vi "EVM_Sweep_record_ALL.vi"() -> ()   [LabVIEW 2023, in "EVM.lvlib"]
uses:
  EVM.lvlib
  Clover_Cell.lvlib
  lib/Keysight/Keysight.lvlib
panel:
  in  "Air_Loss":dbl=8.0
  in  "Cable_Loss":dbl=8.0
  in  "WaitingTime(ms)":u32=1000
  in  "FileNote":string
  in  "TRXmode":u16(ring)=1 items=["QUERY_TELEM_2 (V)"=2, "QUERY_TELEM_1 (H)"=1]
  out "SG Power (dBm)":i32
  in  "Stop Power":i32=8
  in  "Start Power":i32=-40
  in  "SG":refnum<visa-resource-name>="TCPIP0::192.168.100.200::inst0::INSTR"
  in  "SA":refnum<visa-resource-name>="TCPIP0::192.168.100.230::inst0::INSTR"
  in  "AvgTimes":i32=5
  out "Spectrum Data":dbl[](graph)
  out "AiP_8":dbl format="%#2.2f"
  out "AiP_7":dbl format="%#2.2f"
  out "AiP_6":dbl format="%#2.2f"
  out "AiP_5":dbl format="%#2.2f"
  out "AiP_4":dbl format="%#2.2f"
  out "AiP_3":dbl format="%#2.2f"
  out "AiP_2":dbl format="%#2.2f"
  out "AiP_1":dbl format="%#2.2f"
  # "Temperature"
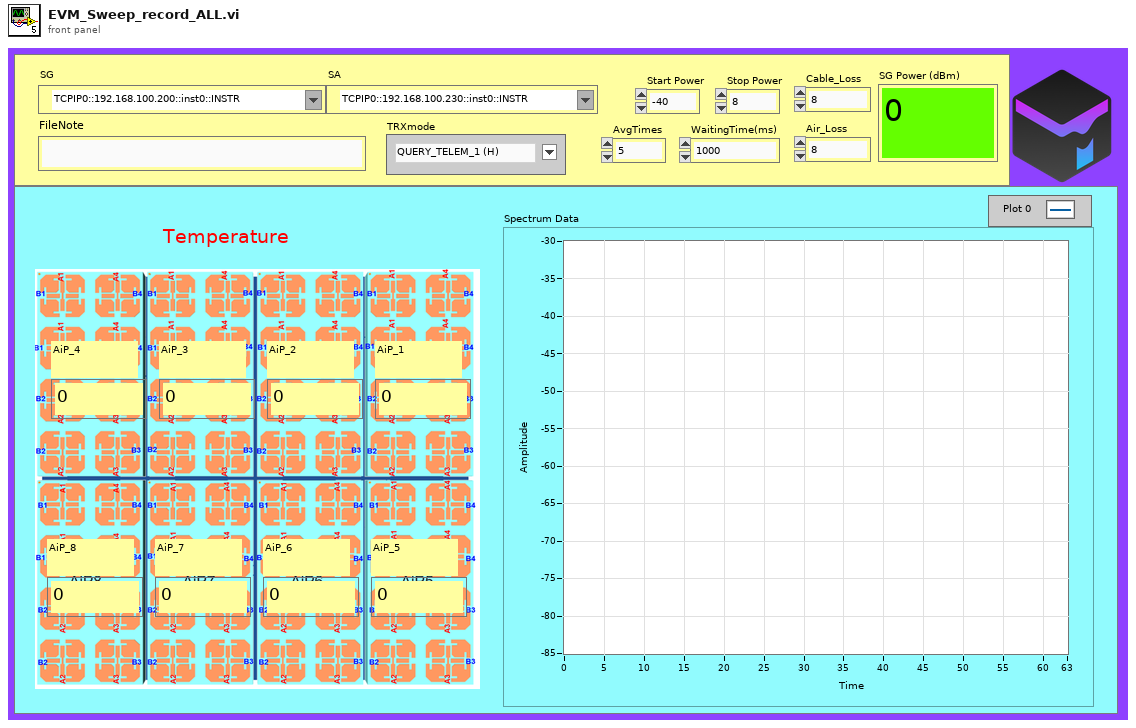
[diagram p1: front panel]
types:
  T1 = cluster{"RMS EVM Avg (dB)":dbl, "RMS EVM Avg (%)":dbl, "Frequency Error Avg (Hz)":dbl, "Avg Burst Power Avg (dBm)":dbl, "Frequency Error Avg (ppm)":dbl}
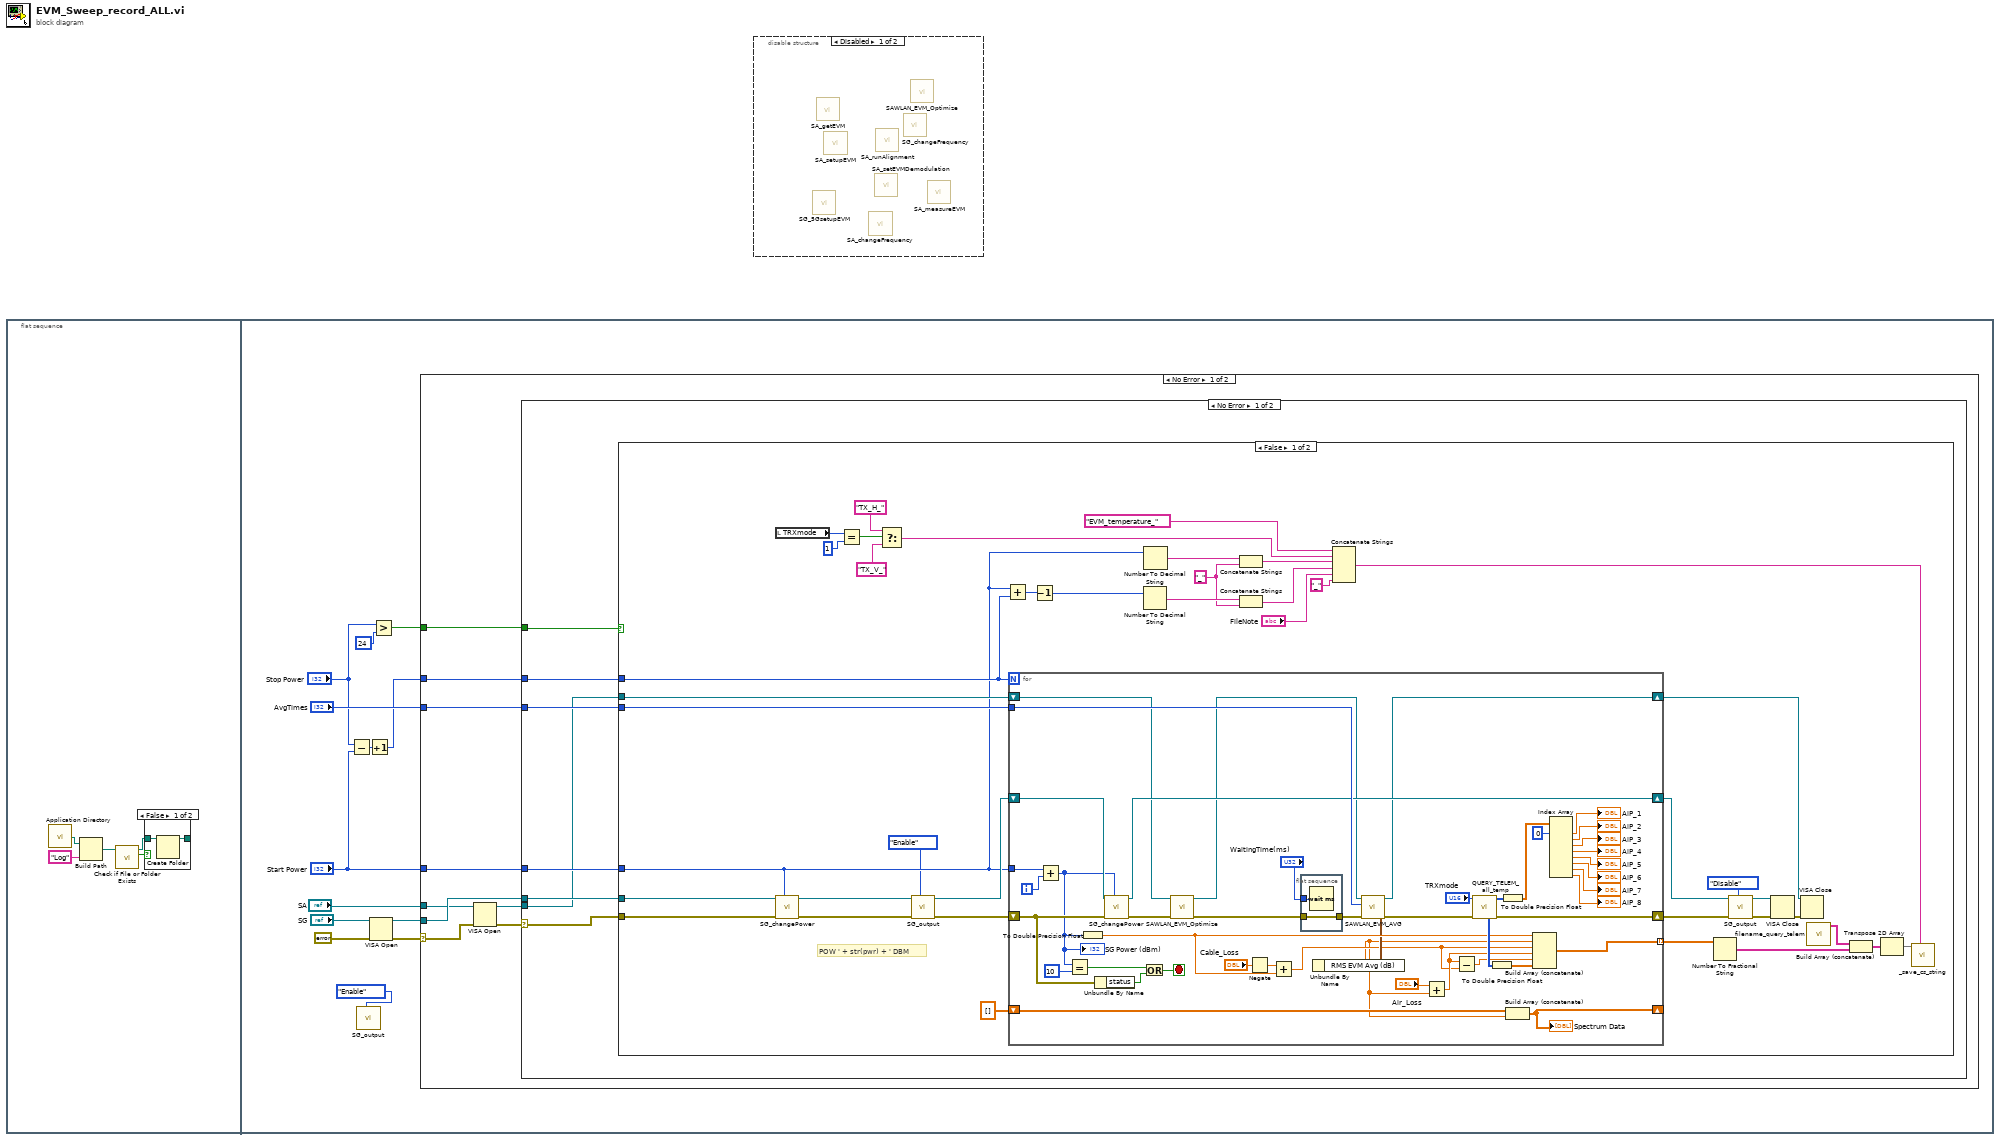
[diagram p0: block diagram]
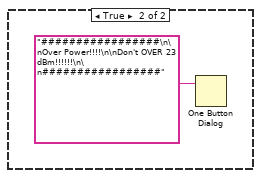
[diagram p4: hidden frame]
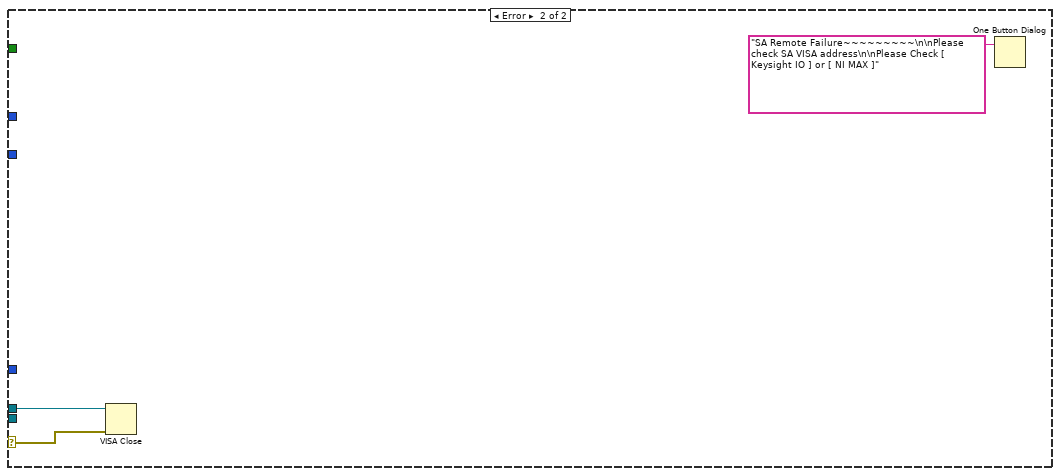
[diagram p5: hidden frame]
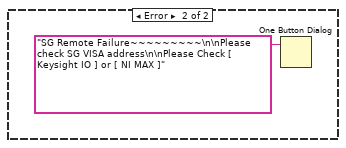
[diagram p6: hidden frame]
diagram:
  n1 = flat-sequence {
    frame #0 {
      n2 = call <vilib>:"Application Directory.vi"() -> ("Application Directory"=w4:path)
      n3 = Build Path(base path=w4, name or relative path="Log") -> (appended path=w1:path)
      n4 = call <vilib>:"Check if File or Folder Exists.vi"("path"=w1) -> ("file or folder exists?"=w3:bool, "dup path"=w2:path)  [unwired: 8 in, 1 out]
      n5 = case shown="False" w3 {
        tunnel: w2 -> [w7 w8]
        tunnel: [w6 w8] -> _
        frame False {
          n6 = Create Folder(path (use dialog)=w7) -> (created path=w6:path)  [unwired: 2 in, 2 out]
        }
        frame True {
        }
      }
    }
    frame #1 {
      n7 = Subtract(x="Stop Power", y="Start Power") -> (x-y=w18:i32)
      n8 = call "SG_output.vi"("Func."=enum16{"Disable", "Enable"}."Enable") -> ()  [unwired: 9 in, 2 out]
      n9 = Increment(x=w18) -> (x+1=w17:i32)
      n10 = VISA Open(error in (no error)=errorcluster {"status"=FALSE, "code"=0, "source"=""}, VISA resource name="SG") -> (VISA resource name=w12:refnum<visa-resource-name>, error out=w10:errorcluster)  [unwired: 3 in]
      n11 = Greater?(x="Stop Power", y=24) -> (0:w21:bool)
      n12 = case shown="No Error" w10 {
        selector: w10 -> [w23 _]
        tunnel: w21 -> [w30 _]
        tunnel: "Start Power" -> [w29 _]
        tunnel: "AvgTimes" -> [w28 _]
        tunnel: w17 -> [w27 _]
        tunnel: w12 -> [w26 _]
        tunnel: "SA" -> [w25 _]
        frame No Error {
          n13 = VISA Open(error in (no error)=w23, VISA resource name=w25) -> (VISA resource name=w24:refnum<visa-resource-name>, error out=w22:errorcluster)  [unwired: 3 in]
          n14 = case shown="No Error" w22 {
            selector: w22 -> [w31 w128]
            tunnel: w30 -> [w37 _]
            tunnel: w29 -> [w36 _]
            tunnel: w28 -> [w35 _]
            tunnel: w27 -> [w34 _]
            tunnel: w26 -> [w33 w129]
            tunnel: w24 -> [w32 _]
            frame No Error {
              n15 = case shown="False" w37 {
                tunnel: w35 -> [w78 _]
                tunnel: w36 -> [w40 _]
                tunnel: w31 -> [w76 _]
                tunnel: w33 -> [w75 _]
                tunnel: w34 -> [w73 _]
                tunnel: w32 -> [w49 _]
                frame False {
                  w65 = "_"
                  # "POW ' + str(pwr) + ' DBM"
                  n16 = local read "TRXmode"() -> (w48:u16)
                  n17 = call "SG_changePower.vi"("dBm"=w40, "error in"=w76, "VISA in"=w75) -> ("error out"=w77:errorcluster, "VISA out"=w74:refnum<visa-resource-name>)  [unwired: 6 in, 1 out]
                  n18 = Equal?(x=w48, y=u16 1) -> (x = y?=w46:bool)
                  n19 = Select(t="TX_H_" ("delimiter (\\t)"), s=w46, f="TX_V_" ("delimiter (\\t)")) -> (s? t:f=w43:string)
                  n20 = call "SG_output.vi"("Func."=enum16{"Disable", "Enable"}."Enable", "error in"=w77, "VISA in"=w74) -> ("error out"=w71:errorcluster, "VISA out"=w72:refnum<visa-resource-name>)  [unwired: 7 in]
                  n21 = Add(x=w40, y=w73) -> (x+y=w69:i32)
                  n22 = for {
                    N: w73 -> [_]
                    tunnel: w78 -> [w124]
                    tunnel: w40 -> [w122]
                    tunnel: [w121] -> w57 mode=indexing
                    shift-right: [w118] -> w70
                    shift-left: w71 -> [w102]
                    shift-right: [w115] -> w62
                    shift-left: w72 -> [w114]
                    shift-right: [w98] -> w50
                    shift-left: w49 -> [w81]
                    shift-right: [w94] -> _
                    shift-left: dbl[] [] -> [w95]
                    i -> [w123]
                    stop <- w101 stop-if-true
                    n23 = Add(x=w122, y=w123) -> (x+y=w84:i32)
                    "SG Power (dBm)" <- w84
                    n24 = Equal?(x=w84, y=10) -> (x = y?=w100:bool)
                    n25 = To Double Precision Float(number=w84) -> (double precision float=w91:dbl)
                    n26 = Unbundle By Name(w102) -> ("status"=w99:bool)
                    n27 = call "SG_changePower.vi"("dBm"=w84, "error in"=w102, "VISA in"=w114) -> ("error out"=w83:errorcluster, "VISA out"=w115:refnum<visa-resource-name>)  [unwired: 6 in, 1 out]
                    n28 = Or(x=w100, y=w99) -> (x .or. y?=w101:bool)
                    n29 = call "SAWLAN_EVM_Optimize.vi"("error in"=w83, "VISA in"=w81) -> ("error out"=w82:errorcluster, "VISA out"=w80:refnum<visa-resource-name>)  [unwired: 8 in]
                    n30 = Negate(x="Cable_Loss") -> (-x=w92:dbl)
                    n31 = Add(x=w92, y=w91) -> (x+y=w86:dbl)
                    n32 = flat-sequence {
                      tunnel: w82 -> [w126]
                      tunnel: [w126] -> w97
                      tunnel: "WaitingTime(ms)" -> [w125]
                      frame #0 {
                        n33 = Wait (ms)(milliseconds to wait=w125) -> ()  [unwired: 1 out]
                      }
                    }
                    n34 = call "SAWLAN_EVM_AVG.vi"("error in (no error)"=w97, "AvgTimes"=w124, "VISA resource name"=w80) -> ("error out"=w119:errorcluster, "VISA resource name out"=w98:refnum<visa-resource-name>, "output"=w89:T1)  [unwired: 6 in]
                    n35 = Unbundle By Name(w89) -> ("RMS EVM Avg (dB)"=w79:dbl)
                    n36 = Add(x="Air_Loss", y=w79) -> (x+y=w87:dbl)
                    n37 = Subtract(x=w87, y=w86) -> (x-y=w85:dbl)
                    n38 = call "QUERY_TELEM_all_temp.vi"("error in"=w119, "TRXmode"="TRXmode") -> ("error out"=w118:errorcluster, "Temp_8pcs"=w117:i32[], "all_data"=w103:i32[])  [unwired: 7 in]
                    n39 = To Double Precision Float(number=w103) -> (double precision float=w88:dbl[])
                    n40 = To Double Precision Float(number=w117) -> (double precision float=w113:dbl[])
                    n41 = Build Array (concatenate)(w95, w79) -> (w94:dbl[])
                    "Spectrum Data" <- w94
                    n42 = Build Array (concatenate)(w91, w79, w86, w87, w85, w88) -> (w121:dbl[])
                    n43 = Index Array(array=w113, index #1=0 ("index")) -> (element #1=→"AiP_1":dbl, element #2=→"AiP_2":dbl, element #3=→"AiP_3":dbl, element #4=→"AiP_4":dbl, element #5=→"AiP_5":dbl, element #6=→"AiP_6":dbl, element #7=→"AiP_7":dbl, element #8=→"AiP_8":dbl)  [unwired: 7 in]
                  }
                  n44 = Decrement(x=w69) -> (x-1=w68:i32)
                  n45 = Number To Decimal String(number=w68) -> (decimal integer string=w66:string)  [unwired: 1 in]
                  n46 = Number To Decimal String(number=w40) -> (decimal integer string=w67:string)  [unwired: 1 in]
                  n47 = Concatenate Strings(w67, w65) -> (w64:string)
                  n48 = Concatenate Strings(w66, w65) -> (w63:string)
                  n49 = Concatenate Strings("EVM_temperature_" ("delimiter (\\t)"), w43, w64, w63, "FileNote", "_") -> (w56:string)
                  n50 = Number To Fractional String(number=w57) -> (F-format string=w58:string[][])  [unwired: 3 in]
                  n51 = call "SG_output.vi"("Func."=enum16{"Disable", "Enable"}."Disable", "error in"=w70, "VISA in"=w62) -> ("error out"=w53:errorcluster, "VISA out"=w52:refnum<visa-resource-name>)  [unwired: 7 in]
                  n52 = VISA Close(VISA resource name=w52, error in (no error)=w53) -> (error out=w51:errorcluster)
                  n53 = VISA Close(VISA resource name=w50, error in (no error)=w51) -> ()  [unwired: 1 out]
                  n54 = call "filename_query_telem.vi"() -> ("appended array"=w54:string[][])  [unwired: 11 in]
                  n55 = Build Array (concatenate)(w54, w58) -> (w59:string[][])
                  n56 = Transpose 2D Array(2D array=w59) -> (transposed array=w55:string[][])
                  n57 = call "_save_cs_string.vi"("FileName"=w56, "Array"=w55) -> ()  [unwired: 9 in, 1 out]
                }
                frame True {
                  n58 = One Button Dialog(message="#################\n\nOver Power!!!!\n\nDon't OVER 23 dBm!!!!!!\n\n#################") -> ()  [unwired: 1 in, 1 out]
                }
              }
            }
            frame Error {
              n59 = VISA Close(VISA resource name=w129, error in (no error)=w128) -> ()  [unwired: 1 out]
              n60 = One Button Dialog(message="SA Remote Failure~~~~~~~~~\n\nPlease check SA VISA address\n\nPlease Check [ Keysight IO ] or [ NI MAX ]") -> ()  [unwired: 1 in, 1 out]
            }
          }
        }
        frame Error {
          n61 = One Button Dialog(message="SG Remote Failure~~~~~~~~~\n\nPlease check SG VISA address\n\nPlease Check [ Keysight IO ] or [ NI MAX ]") -> ()  [unwired: 1 in, 1 out]
        }
      }
    }
  }
  n62 = disable-structure shown="Disabled" {
    frame Disabled {
      n63 = call "SG_5GsetupEVM.vi"() -> ()  [unwired: 9 in, 3 out]
      n64 = call "SA_getEVM.vi"() -> ()  [unwired: 9 in, 3 out]
      n65 = call "SA_setupEVM.vi"() -> ()  [unwired: 9 in, 3 out]
      n66 = call "SA_changeFrequency.vi"() -> ()  [unwired: 9 in, 3 out]
      n67 = call "SA_setEVMDemodulation.vi"() -> ()  [unwired: 9 in, 3 out]
      n68 = call "SA_runAlignment.vi"() -> ()  [unwired: 9 in, 3 out]
      n69 = call "SG_changeFrequency.vi"() -> ()  [unwired: 9 in, 3 out]
      n70 = call "SAWLAN_EVM_Optimize.vi"() -> ()  [unwired: 10 in, 2 out]
      n71 = call "SA_measureEVM.vi"() -> ()  [unwired: 9 in, 3 out]
    }
    frame Enabled {
    }
  }
